vi "punto3 10sampls.vi"() -> ()   [LabVIEW 2025]
uses:
  <vilib>/express/express analysis/Spectral/Block/exnSpectralBlock spectral measurements peak poly.vi
  <vilib>/express/express analysis/Spectral/Block/exnSpectralBlock spectral measurements peak DDT.vi
  <vilib>/express/express analysis/Spectral/XNode/ExpressSpectralMeasurementsBlockNode.xnode
panel:
  out "DFT":dynamicdata(graph)
  out "sin":dynamicdata(graph)
  in  "#s":i32=1000
  in  "Fs":dbl=1000.0
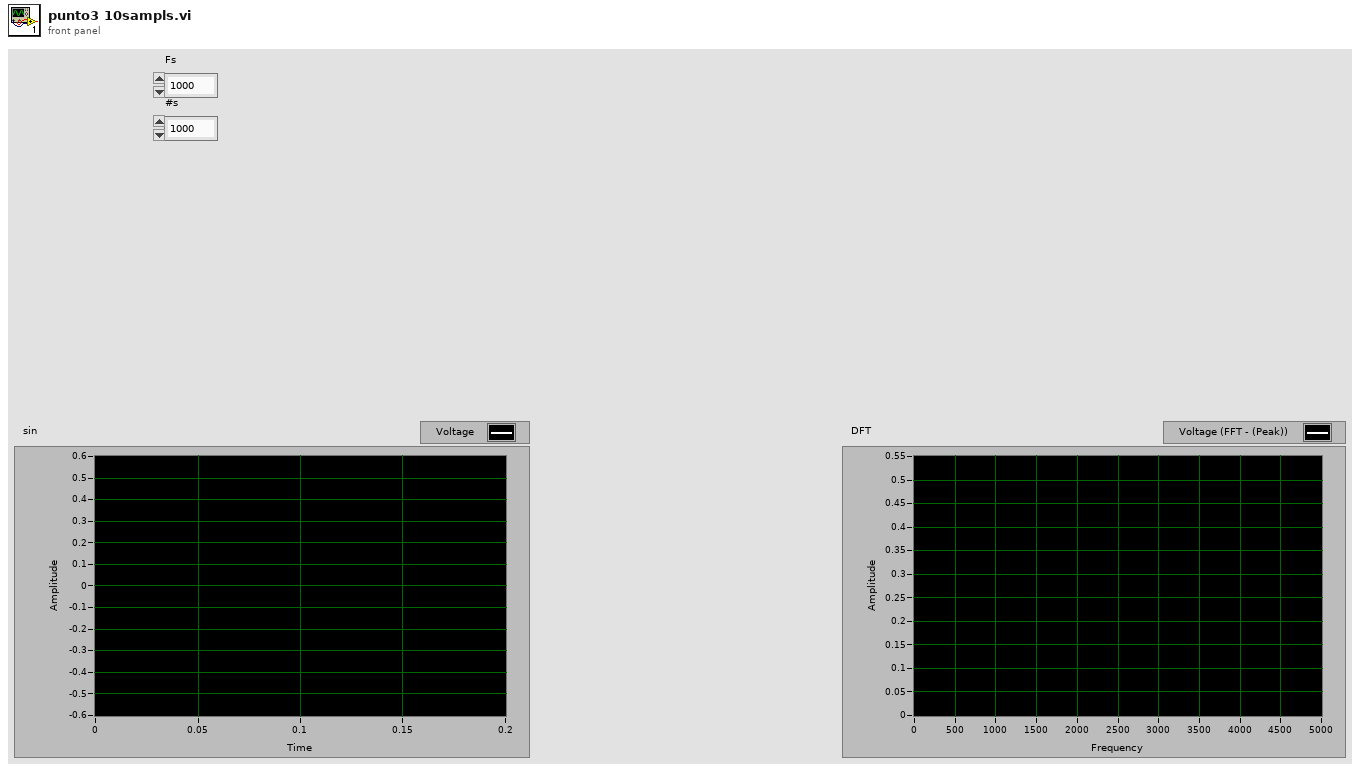
[diagram p1: front panel]
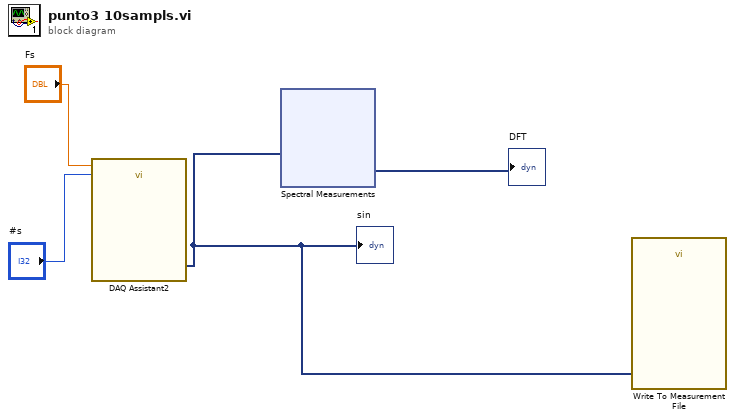
[diagram p0: block diagram]
diagram:
  n1 = call "DAQ Assistant2"("rate"="Fs", "number of samples"="#s") -> ("data"=w1:dynamicdata)  [unwired: 15 in, 2 out]
  "sin" <- w1
  n2 = xnode "Spectral Measurements"("Signals"=w1) -> ("FFT - (Peak)"=→"DFT":dynamicdata)  [unwired: 1 in, 2 out]
  n3 = call "Write To Measurement File"("Signals"=w1) -> ()  [unwired: 16 in, 3 out]
